vi "LinkCameras.vi"(0 "L_Image":T2, 1 "Green or Sat Range":cluster{"Lower value":i32, "Upper value":i32}={"Lower value"=0, "Upper value"=255}, 2 "Red or Hue Range":cluster{"Lower value":i32, "Upper value":i32}={"Lower value"=80, "Upper value"=100}, 3 "R_Image":T2, 4 "Blue or Luma or Val or Inten Range":cluster{"Lower value":i32, "Upper value":i32}={"Lower value"=20, "Upper value"=120}) -> (5 "L_Image Out":T2, 6 "TargetMatch":T1(array[cluster]), 7 "R_Image Out":T2)   [LabVIEW 2011]
uses:
  <vilib>/vision/Image Controls.llb/IMAQ Image.ctl
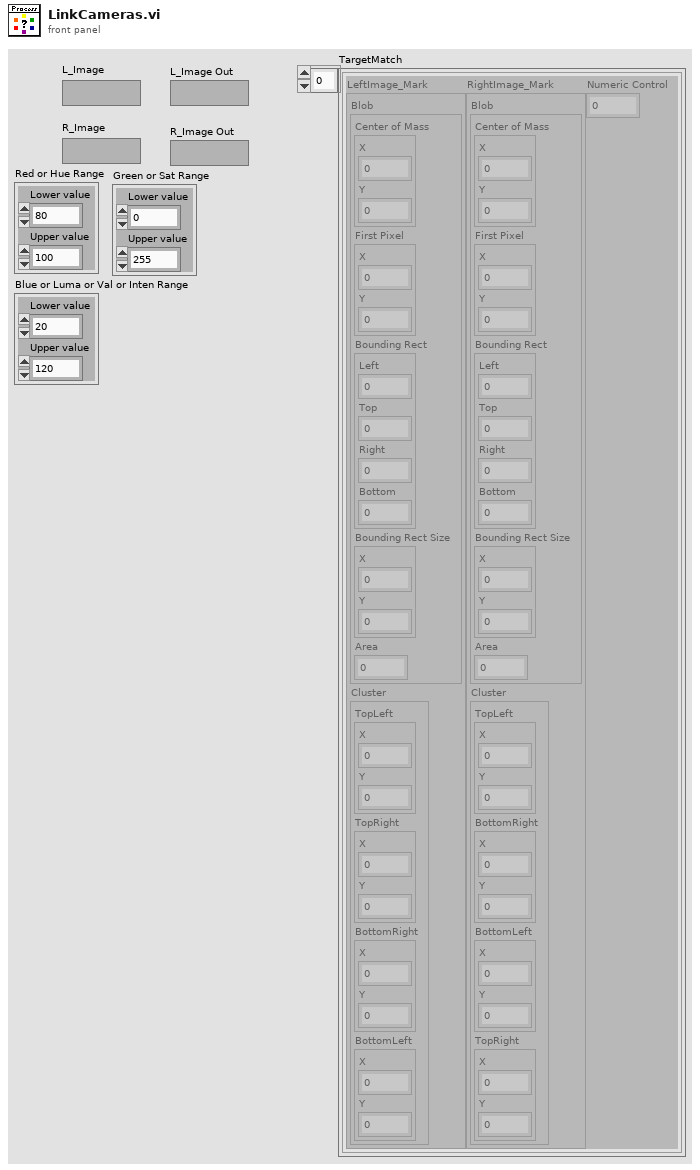
[diagram p1: front panel]
types:
  T1 = cluster{"LeftImage_Mark":cluster{"Blob":cluster{"Center of Mass":cluster{"X":dbl, "Y":dbl}, "First Pixel":cluster{"X":dbl, "Y":dbl}, "Bounding Rect":cluster{"Left":dbl, "Top":dbl, "Right":dbl, "Bottom":dbl}, "Bounding Rect Size":cluster{"X":dbl, "Y":dbl}, "Area":dbl}, "Cluster":cluster{"TopLeft":cluster{"X":dbl, "Y":dbl}, "TopRight":cluster{"X":dbl, "Y":dbl}, "BottomRight":cluster{"X":dbl, "Y":dbl}, "BottomLeft":cluster{"X":dbl, "Y":dbl}}}, "RightImage_Mark":cluster{"Blob":cluster{"Center of Mass":cluster{"X":dbl, "Y":dbl}, "First Pixel":cluster{"X":dbl, "Y":dbl}, "Bounding Rect":cluster{"Left":dbl, "Top":dbl, "Right":dbl, "Bottom":dbl}, "Bounding Rect Size":cluster{"X":dbl, "Y":dbl}, "Area":dbl}, "Cluster":cluster{"TopLeft":cluster{"X":dbl, "Y":dbl}, "BottomRight":cluster{"X":dbl, "Y":dbl}, "BottomLeft":cluster{"X":dbl, "Y":dbl}, "TopRight":cluster{"X":dbl, "Y":dbl}}}, "Numeric Control":dbl}[]
  T2 = typedef "IMAQ Image.ctl" = refnum<image>
  T3 = typedef "Image Type" = u32
  T4 = cluster{"Start Point":cluster{"X":sgl, "Y":sgl}, "End Point":cluster{"X":sgl, "Y":sgl}, "Length":dbl, "Orientation":dbl, "Score":dbl}[]
  T5 = cluster{"Center of Mass":cluster{"X":dbl, "Y":dbl}, "First Pixel":cluster{"X":dbl, "Y":dbl}, "Bounding Rect":cluster{"Left":dbl, "Top":dbl, "Right":dbl, "Bottom":dbl}, "Bounding Rect Size":cluster{"X":dbl, "Y":dbl}, "Area":dbl}[]
  T6 = cluster{"Blob":cluster{"Center of Mass":cluster{"X":dbl, "Y":dbl}, "First Pixel":cluster{"X":dbl, "Y":dbl}, "Bounding Rect":cluster{"Left":dbl, "Top":dbl, "Right":dbl, "Bottom":dbl}, "Bounding Rect Size":cluster{"X":dbl, "Y":dbl}, "Area":dbl}, cluster{"TopLeft":cluster{"X":dbl, "Y":dbl}, "TopRight":cluster{"X":dbl, "Y":dbl}, "BottomRight":cluster{"X":dbl, "Y":dbl}, "BottomLeft":cluster{"X":dbl, "Y":dbl}}}[]
  T7 = cluster{"Blob":cluster{"Center of Mass":cluster{"X":dbl, "Y":dbl}, "First Pixel":cluster{"X":dbl, "Y":dbl}, "Bounding Rect":cluster{"Left":dbl, "Top":dbl, "Right":dbl, "Bottom":dbl}, "Bounding Rect Size":cluster{"X":dbl, "Y":dbl}, "Area":dbl}, "Cluster":cluster{"TopLeft":cluster{"X":dbl, "Y":dbl}, "TopRight":cluster{"X":dbl, "Y":dbl}, "BottomRight":cluster{"X":dbl, "Y":dbl}, "BottomLeft":cluster{"X":dbl, "Y":dbl}}}
  T8 = cluster{"Blob":cluster{"Center of Mass":cluster{"X":dbl, "Y":dbl}, "First Pixel":cluster{"X":dbl, "Y":dbl}, "Bounding Rect":cluster{"Left":dbl, "Top":dbl, "Right":dbl, "Bottom":dbl}, "Bounding Rect Size":cluster{"X":dbl, "Y":dbl}, "Area":dbl}, "Cluster":cluster{"TopLeft":cluster{"X":dbl, "Y":dbl}, "BottomRight":cluster{"X":dbl, "Y":dbl}, "BottomLeft":cluster{"X":dbl, "Y":dbl}, "TopRight":cluster{"X":dbl, "Y":dbl}}}
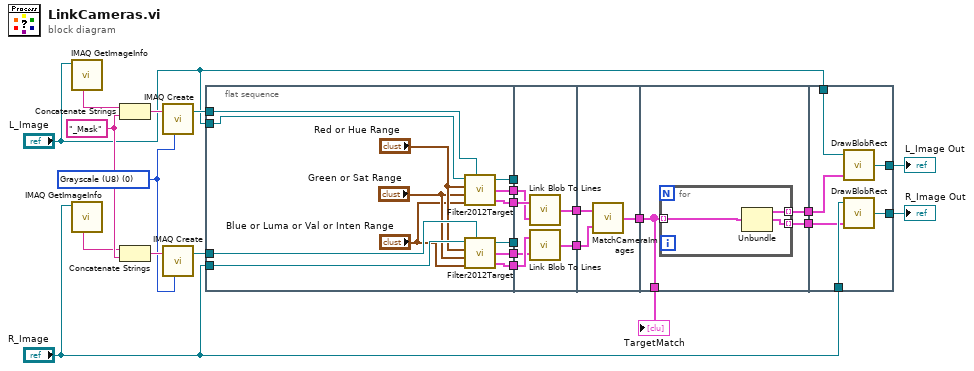
[diagram p0: block diagram]
diagram:
  w13 = T3 0 items=["Grayscale (U8)", "Grayscale (I16)", "Grayscale (SGL)", "Complex (CSG)", "RGB (U32)", "HSL (U32)", "RGB (U64)", "Grayscale (U16)"] ("Image Type")
  w15 = "_Mask" ("string")
  n1 = call "IMAQ GetImageInfo"("Image"="L_Image") -> ("Image Name"=w18:string)  [unwired: 3 in, 7 out]
  n2 = call "IMAQ GetImageInfo"("Image"="R_Image") -> ("Image Name"=w14:string)  [unwired: 3 in, 7 out]
  n3 = Concatenate Strings(w18, w15) -> (w19:string)
  n4 = Concatenate Strings(w14, w15) -> (w17:string)
  n5 = call "IMAQ Create"("Image Name"=w19, "Image Type"=w13) -> ("New Image"=w20:T2)  [unwired: 3 in, 1 out]
  n6 = call "IMAQ Create"("Image Name"=w17, "Image Type"=w13) -> ("New Image"=w16:T2)  [unwired: 3 in, 1 out]
  n7 = flat-sequence {
    tunnel: "R_Image" -> [w33]
    tunnel: "L_Image" -> [w35]
    tunnel: [w34] -> w22
    tunnel: [w32] -> w21
    tunnel: w20 -> [w37]
    tunnel: w16 -> [w36]
    tunnel: [w31] -> w12
    tunnel: [w30] -> w11
    tunnel: [w29] -> w10
    tunnel: [w28] -> w9
    tunnel: [w43] -> w24
    tunnel: [w42] -> w23
    tunnel: w22 -> [_]
    tunnel: w21 -> [_]
    tunnel: w12 -> [w41]
    tunnel: w11 -> [w40]
    tunnel: w10 -> [w39]
    tunnel: w9 -> [w38]
    tunnel: w24 -> [w45]
    tunnel: w23 -> [w46]
    tunnel: [w44] -> w8
    tunnel: w8 -> [w49]
    tunnel: [w49] -> w1
    tunnel: [w48] -> w5
    tunnel: [w47] -> w4
    tunnel: "L_Image" -> [w58]
    tunnel: "R_Image" -> [w57]
    tunnel: w5 -> [w56]
    tunnel: w4 -> [w55]
    tunnel: [w54] -> w3
    tunnel: [w53] -> w2
    frame #0 {
      n8 = call "Filter2012Target.vi"("Image In"=w35, "Red or Hue Range"="Red or Hue Range", "Green or Sat Range"="Green or Sat Range", "Blue or Luma or Val or Inten Range"="Blue or Luma or Val or Inten Range", "Image Dst"=w37) -> ("Image Out"=w34:T2, "Lines Calibrated"=w30:T4, "Blob Array"=w31:T5)
      n9 = call "Filter2012Target.vi"("Image In"=w33, "Red or Hue Range"="Red or Hue Range", "Green or Sat Range"="Green or Sat Range", "Blue or Luma or Val or Inten Range"="Blue or Luma or Val or Inten Range", "Image Dst"=w36) -> ("Image Out"=w32:T2, "Lines Calibrated"=w28:T4, "Blob Array"=w29:T5)
    }
    frame #1 {
      n10 = call "Link Blob To Lines.vi"("Lines Calibrated"=w40, "Blob Array"=w41) -> ("TargetArray"=w42:T6)
      n11 = call "Link Blob To Lines.vi"("Lines Calibrated"=w38, "Blob Array"=w39) -> ("TargetArray"=w43:T6)
    }
    frame #2 {
      n12 = call "MatchCameraImages.vi"("R_TargetArray"=w45, "L_TargetArray"=w46) -> ("TargetMatch"=w44:T1)
    }
    frame #3 {
      n13 = for {
        tunnel: w49 -> [w52] mode=indexing
        tunnel: [w51] -> w47 mode=indexing
        tunnel: [w50] -> w48 mode=indexing
        n14 = Unbundle(w52) -> ("LeftImage_Mark"=w51:T7, "RightImage_Mark"=w50:T8)  [unwired: 1 out]
      }
    }
    frame #4 {
      n15 = call "DrawBlobRect.vi"("BlobLineDataArray"=w55, "Src In"=w58) -> ("Image Out"=w54:T2)  [unwired: 1 in]
      n16 = call "DrawBlobRect.vi"("BlobLineDataArray"=w56, "Src In"=w57) -> ("Image Out"=w53:T2)  [unwired: 1 in]
    }
  }
  "L_Image Out" <- w3
  "R_Image Out" <- w2
  "TargetMatch" <- w1
